vi "main.vi"() -> ()   [LabVIEW 2024]
uses:
  kontrakt.ctl
  <vilib>/addons/_JKI.lib/REST Client/classes/REST Client/REST Client.lvclass
  measure_data.ctl
panel:
  out "Response body":string
  in  "auto read":bool
  out "Waveform Graph 2":dbl[](graph)
  in  "Base URL":string
  in  "connect":bool
  in  "measure":bool
  in  "exit":bool
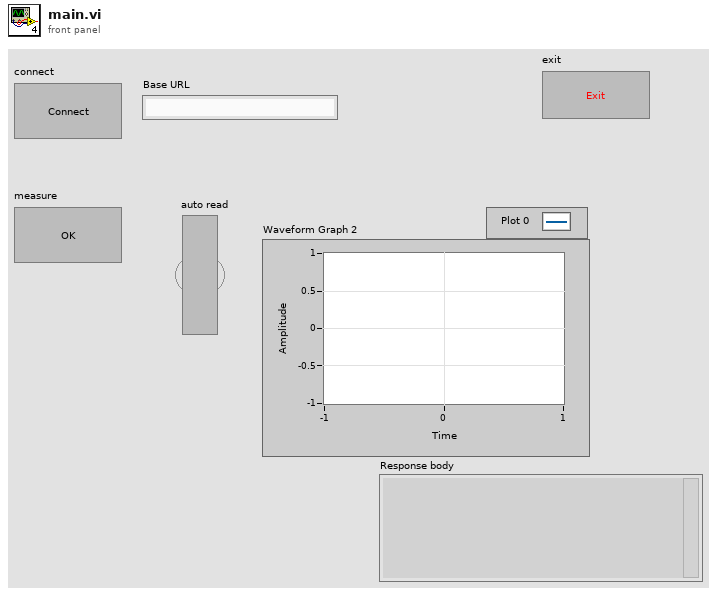
[diagram p1: front panel]
types:
  T1 = cluster{"polaczenie":refnum<class "REST Client.lvclass">, "dane":dbl[], "flag":bool, "text":string}
  T2 = typedef "kontrakt.ctl" = cluster{"akcja":enum16{"get_measure", "exit_program", "init_session", "close_session", "set_flag"}, "parametry":variant}
  T3 = enum16{"get_measure", "exit_program", "init_session", "close_session", "set_flag"}
  T4 = typedef "measure_data.ctl" = cluster{"value":dbl, "String":string}
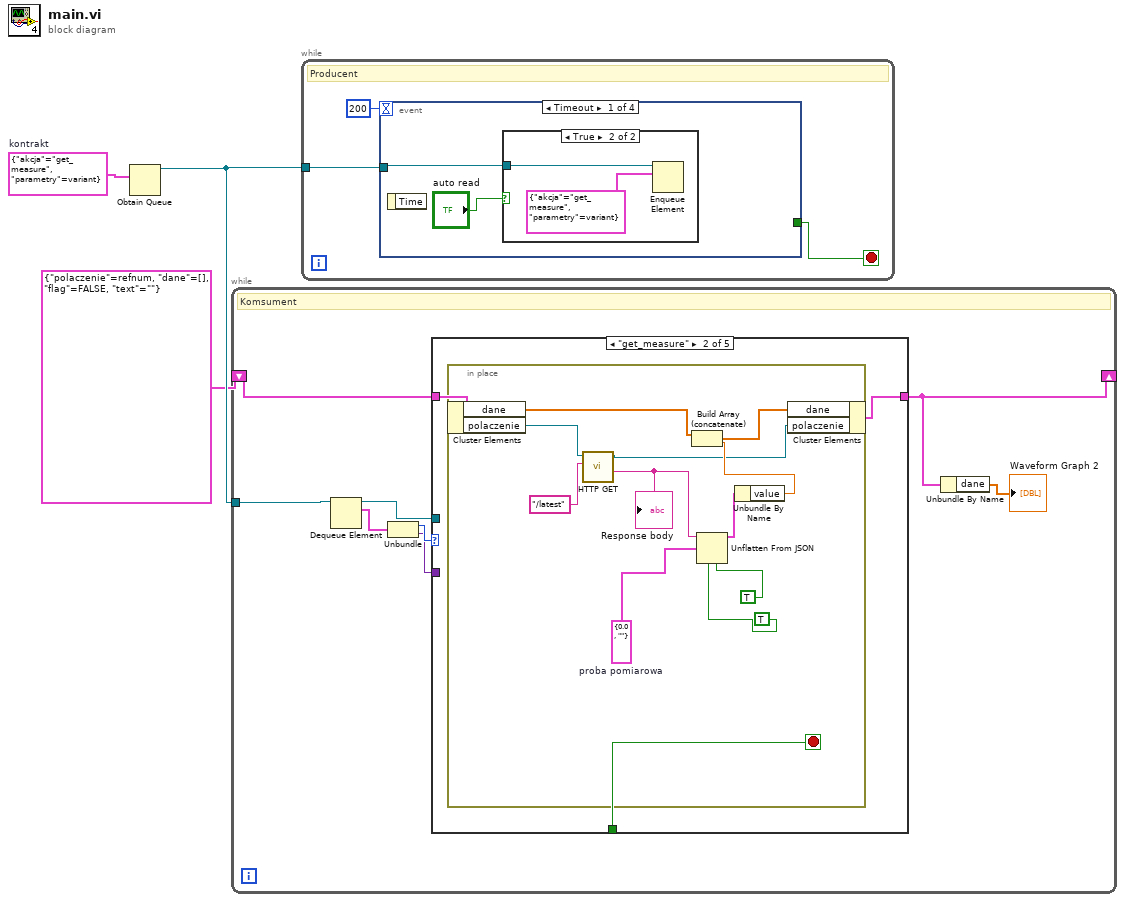
[diagram p0: block diagram]
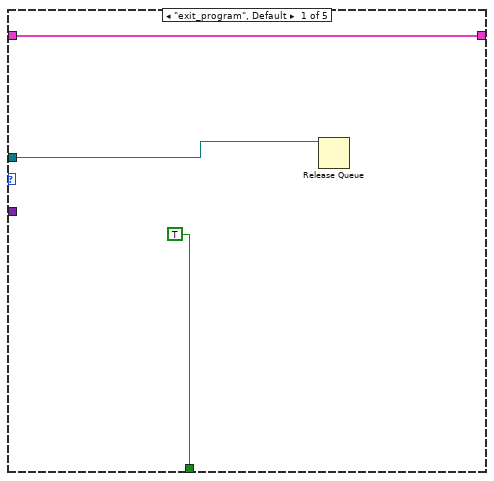
[diagram p2: hidden frame]
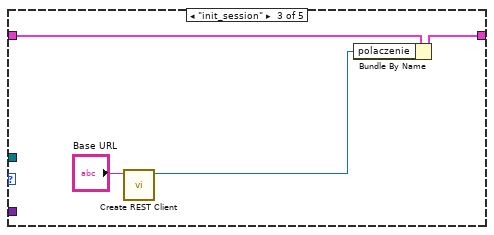
[diagram p3: hidden frame]
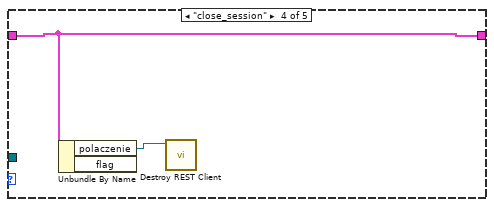
[diagram p4: hidden frame]
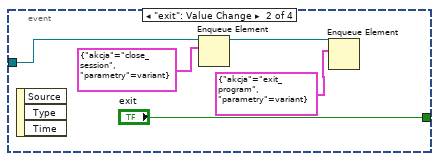
[diagram p7: hidden frame]
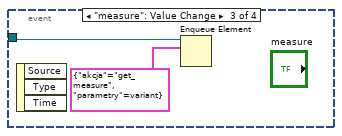
[diagram p8: hidden frame]
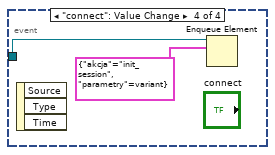
[diagram p9: hidden frame]
diagram:
  w2 = T2 {"akcja"=enum."get_measure", "parametry"=variant}  # kontrakt
  n1 = Obtain Queue(element data type=w2) -> (queue out=w3:refnum<queue>)  [unwired: 4 in, 2 out]
  n2 = while {
    tunnel: w3 -> [w12]
    shift-right: [w5] -> _
    shift-left: T1 {"polaczenie"=refnum, "dane"=[], "flag"=FALSE, "text"=""} -> [w6]
    stop <- w7 stop-if-true
    # "Komsument"
    n3 = Dequeue Element(queue=w12) -> (queue out=w8:refnum<queue>, element=w11:T2)  [unwired: 2 in, 2 out]
    n4 = Unbundle(w11) -> ("akcja"=w10:T3, "parametry"=w9:variant)
    n5 = case shown="\"get_measure\"" w10 {
      tunnel: w9 -> [_ _ _ _ _]
      tunnel: w8 -> [w15 _ _ _ _]
      tunnel: [TRUE _ _ _ _] -> w7
      tunnel: w6 -> [w13 w17 w31 w34 w35]
      tunnel: [w13 w16 w30 w34 w35] -> w5
      frame "exit_program", Default {
        n6 = Release Queue(queue=w15) -> ()  [unwired: 2 in, 3 out]
      }
      frame "get_measure" {
        n7 = in-place "In Place Element Structure" {
          w20 = T4 {"value"=0.0, "String"=""}  # proba pomiarowa
          n8 = in-place-cluster #1(w17) -> ("dane"=w24:dbl[], "polaczenie"=w22:refnum<class "REST Client.lvclass">)
          n9 = call-dynamic "HTTP GET.vi"("Path"="/latest", "REST Client in"=w22) -> ("Response body"=w28:string, "REST Client out"=w21:refnum<class "REST Client.lvclass">)  [unwired: 4 in, 4 out]
          "Response body" <- w28
          n10 = Unflatten From JSON(JSON string=w28, type and defaults=w20, default null elements? (F)=TRUE, strict validation? (F)=TRUE) -> (value=w27:T4)  [unwired: 3 in, 1 out]
          n11 = Unbundle By Name(w27) -> ("value"=w26:dbl)
          n12 = Build Array (concatenate)(w24, w26) -> (w23:dbl[])
          n13 = in-place-cluster #1("dane"=w23, "polaczenie"=w21) -> (w16:T1)
        }
      }
      frame "init_session" {
        n14 = call <vilib>:"Create REST Client.vi"("Base URL"="Base URL") -> ("REST Client out"=w29:refnum<class "REST Client.lvclass">)  [unwired: 9 in, 1 out]
        n15 = Bundle By Name(cluster=w31, "polaczenie"=w29) -> (w30:T1)
      }
      frame "close_session" {
        n16 = Unbundle By Name(w34) -> ("polaczenie"=w33:refnum<class "REST Client.lvclass">)  [unwired: 1 out]
        n17 = call-dynamic "Destroy REST Client.vi"("REST Client in"=w33) -> ()  [unwired: 10 in, 1 out]
      }
      frame "set_flag" {
      }
    }
    n18 = Unbundle By Name(w5) -> ("dane"=→"Waveform Graph 2":dbl[])
  }
  n19 = while {
    tunnel: w3 -> [w38]
    stop <- w37 stop-if-true
    # "Producent"
    n20 = event shown="[0] Timeout" {
      selector: _ -> [_ _ _ _]
      dyn-events: _ -> [_ _ _ _]
      timeout: 200 -> [_ _ _ _]
      tunnel: w38 -> [w40 w46 w49 w51]
      tunnel: [_ "exit" _ _] -> w37
      event Timeout {
        n21 = event-data() -> ()  [unwired: 1 in, 1 out]
        n22 = case shown="True" "auto read" {
          tunnel: w40 -> [_ w42]
          frame False {
          }
          frame True {
            n23 = Enqueue Element(queue=w42, element=T2 {"akcja"=enum."get_measure", "parametry"=variant}) -> ()  [unwired: 2 in, 3 out]
          }
        }
      }
      event "exit": Value Change {
        n24 = event-data() -> ()  [unwired: 1 in, 3 out]
        n25 = Enqueue Element(queue=w46, element=T2 {"akcja"=enum."close_session", "parametry"=variant}) -> (queue out=w44:refnum<queue>)  [unwired: 2 in, 2 out]
        n26 = Enqueue Element(queue=w44, element=T2 {"akcja"=enum."exit_program", "parametry"=variant}) -> ()  [unwired: 2 in, 3 out]
      }
      event "measure": Value Change {
        n27 = event-data() -> ()  [unwired: 1 in, 3 out]
        n28 = Enqueue Element(queue=w49, element=T2 {"akcja"=enum."get_measure", "parametry"=variant}) -> ()  [unwired: 2 in, 3 out]
      }
      event "connect": Value Change {
        n29 = event-data() -> ()  [unwired: 1 in, 3 out]
        n30 = Enqueue Element(queue=w51, element=T2 {"akcja"=enum."init_session", "parametry"=variant}) -> ()  [unwired: 2 in, 3 out]
      }
    }
  }
